vi "Superimpose Fiducial Indicator.vi"(6 "Marker Color":u32(colorbox)=16711680, 7 "size":i32=20, 8 "error in":errorcluster, 10 "Fiducial Image Coordinates":refnum<class "Vec3d Class.lvclass">, 11 "Image In":T1) -> (0 "error out":errorcluster, 3 "Image Out":T1)   [LabVIEW 2011]
uses:
  <vilib>/vision/Image Controls.llb/IMAQ Image.ctl
  Vec3d Class/Vec3d Class.lvclass
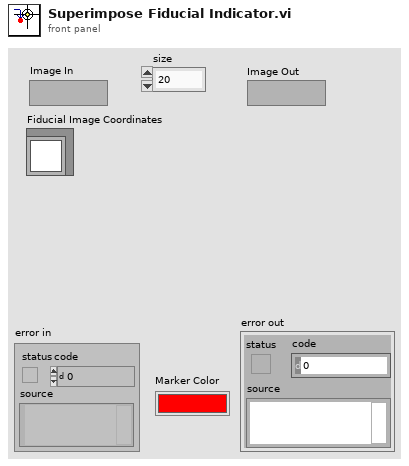
[diagram p1: front panel]
types:
  T1 = typedef "IMAQ Image.ctl" = refnum<image>
  T2 = cluster{"Left":i32, "Top":i32, "Right":i32, "Bottom":i32}
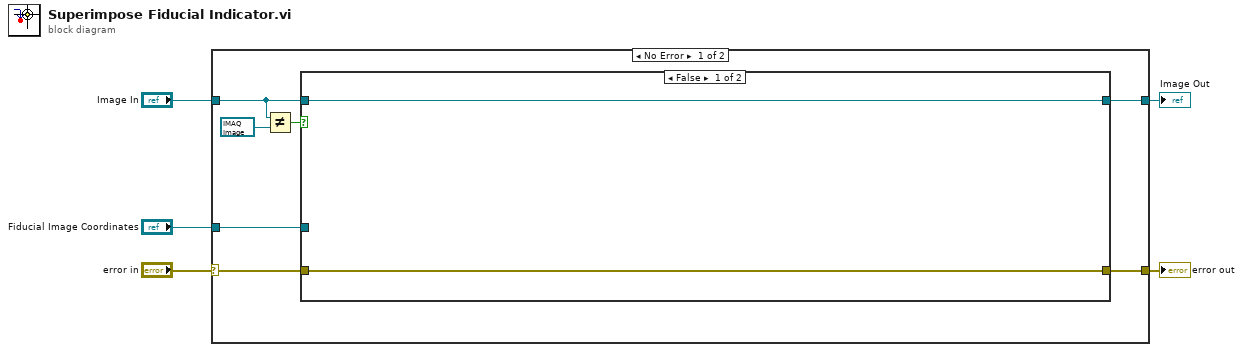
[diagram p0: block diagram]
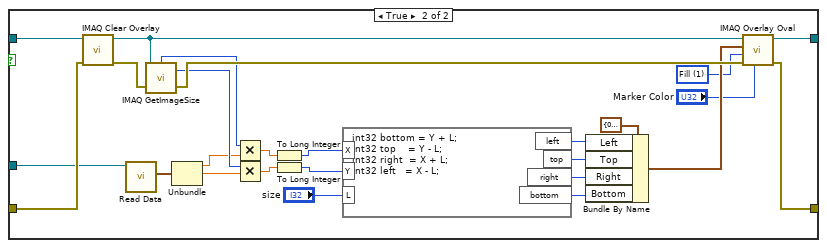
[diagram p2: hidden frame]
diagram:
  n1 = case shown="No Error" "error in" {
    selector: "error in" -> [w12 w42]
    tunnel: "Image In" -> [w7 w41]
    tunnel: [w9 w42] -> w3
    tunnel: "Fiducial Image Coordinates" -> [w11 _]
    tunnel: [w10 w41] -> w1
    frame No Error {
      n2 = Not Equal?(x=w7, y=T1 refnum ("Image In")) -> (x != y?=w6:bool)
      n3 = case shown="False" w6 {
        tunnel: w7 -> [w14 w40]
        tunnel: w12 -> [w13 w39]
        tunnel: w11 -> [_ w36]
        tunnel: [w14 w23] -> w10
        tunnel: [w13 w22] -> w9
        frame False {
        }
        frame True {
          w21 = u32 1 items=["Frame", "Fill"] ("Drawing Mode (Frame)")
          n4 = call "IMAQ Clear Overlay"("error in (no error)"=w39, "Image"=w40) -> ("error out"=w38:errorcluster, "Image Out"=w37:T1)  [unwired: 8 in]
          n5 = call-dynamic "Read Data.vi"("Vec3d Class in"=w36) -> ("Data"=w33:cluster{"X":dbl, "Y":dbl, "Z":dbl})  [unwired: 8 in, 2 out]
          n6 = call "IMAQ GetImageSize"("Image"=w37, "error in (no error)"=w38) -> ("Y Resolution"=w32:i32, "X Resolution"=w31:i32, "error out"=w35:errorcluster)  [unwired: 2 in]
          n7 = Unbundle(w33) -> ("X"=w19:dbl, "Y"=w20:dbl)  [unwired: 1 out]
          n8 = Multiply(x=w31, y=w19) -> (x*y=w18:dbl)
          n9 = Multiply(x=w32, y=w20) -> (x*y=w17:dbl)
          n10 = To Long Integer(number=w18) -> (32bit integer=w16:i32)
          n11 = To Long Integer(number=w17) -> (32bit integer=w15:i32)
          n12 = formula code="int32 bottom = Y + L;\nint32 top    = Y - L;\nint32 right  = X + L;\nint32 left   = X - L;"("X"=w16, "Y"=w15, "L"="size") -> ("left"=w30:i32, "top"=w29:i32, "right"=w28:i32, "bottom"=w27:i32)
          n13 = Bundle By Name(cluster=T2 {"Left"=0, "Top"=0, "Right"=0, "Bottom"=0} ("Bounding Rectangle"), "Left"=w30, "Top"=w29, "Right"=w28, "Bottom"=w27) -> (w26:T2)
          n14 = call "IMAQ Overlay Oval"("Color"="Marker Color", "error in (no error)"=w35, "Drawing Mode (Frame)"=w21, "Bounding Rectangle"=w26, "Image"=w37) -> ("error out"=w22:errorcluster, "Image Out"=w23:T1)  [unwired: 5 in]
        }
      }
    }
    frame Error {
    }
  }
  "error out" <- w3
  "Image Out" <- w1
